vi "Case_Structure.vi"() -> ()   [LabVIEW 2016, in "EV3Group10.lvrbt"]
uses:
  EV3Group10.lvrbt
  <vilib>/NXT/Block Support/NXT_InputPort.ctl
  <vilib>/NXT/Block Support/NXT_OutputPort.ctl
  <vilib>/NXT/Dual Mode Library/Sensors/EV3_Ultrasonic_CM.vi
  <vilib>/NXT/NXTIO Xnodes/NXTIONodeSubVIs/NXTMoveMotors.vi
  <vilib>/NXT/NXTIO Xnodes/NXTIONodeSubVIs/NXTStopMotors.vi
  <vilib>/NXT/Subs/LVHSConnector.ctl
  <vilib>/NXT/NXTIO Xnodes/AddressXNode/NXTIOAddress.xnode
  <vilib>/NXT/NXTIO Xnodes/NXTIOXNode/NXTIO.xnode
  <vilib>/NXT/LegoClasses/BrickReference/BrickReference.lvclass
panel:
  out "Numerisch":dbl
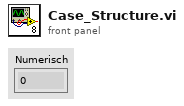
[diagram p1: front panel]
types:
  T1 = typedef "NXT_InputPort.ctl" = u32
  T2 = typedef "NXT_OutputPort.ctl" = u8
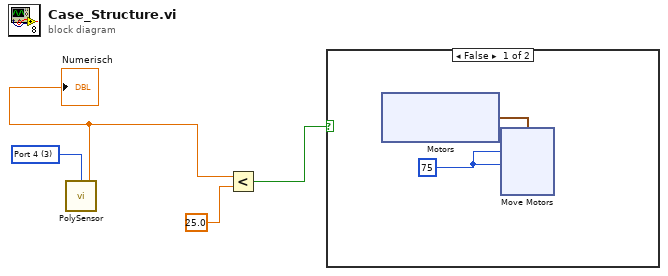
[diagram p0: block diagram]
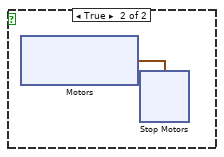
[diagram p2: hidden frame]
diagram:
  w4 = T1 3 items=["Port 1", "Port 2", "Port 3", "Port 4"] ("Port (Port 1)")
  n1 = call-poly <vilib>:"PolySensor.vi"("Port (Port 1)"=w4) -> ("Centimeters"=w1:sgl)  [unwired: 2 in, 1 out]
  "Numerisch" <- w1
  n2 = Less?(x=w1, y=25.0) -> (x < y?=w2:bool)
  n3 = case shown="False" w2 {
    frame False {
      w5 = i8 75 ("Power/Speed 1")
      n4 = xnode "Motors"() -> ("Motor"=w6:cluster{"Port":T2, "Port":T2})
      n5 = xnode "Move Motors"("Power/Speed 2"=w5, "Power/Speed 1"=w5, "Motors"=w6) -> ()  [unwired: 1 in, 1 out]
    }
    frame True {
      n6 = xnode "Motors"() -> ("Motor"=w16:cluster{"Port":T2, "Port":T2})
      n7 = xnode "Stop Motors"("Motors"=w16) -> ()  [unwired: 1 in, 1 out]
    }
  }
